vi "ToDatagram.vi"(8 "error in (no error)":errorcluster, 10 "messageID":u16, 11 "PublishReceivedMqttMsg in":refnum<class "PublishReceivedMqttMsg.lvclass">) -> (0 "error out":errorcluster, 2 "Datagram":u8[](array[numeric]), 3 "PublishReceivedMqttMsg out":refnum<class "PublishReceivedMqttMsg.lvclass">)   [LabVIEW 2020, in "PublishReceivedMqttMsg.lvclass"]
uses:
  PublishReceivedMqttMsg.lvclass
  PublishReceivedMqttMsg.lvclass/PublishReceivedMqttMsg.ctl
  mqttTypedef/MessageType.ctl
  mqttTypedef/QosLevel.ctl
  MQTT Client.lvclass
  BaseMqttMsg.lvclass
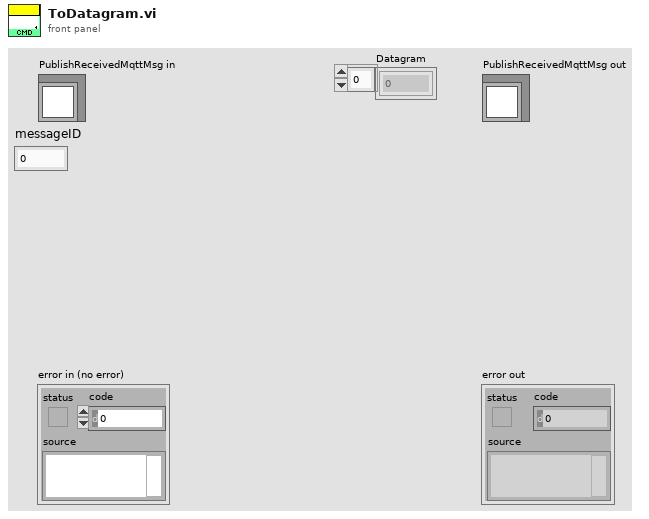
[diagram p1: front panel]
types:
  T1 = typedef "MQTT Client.lvclass/QosLevel.ctl" = enum8{"At most once", "At least once", "Exactly once", "Reserved"}
  T2 = typedef "MQTT Client.lvclass/MessageType.ctl" = enum32{"Reserved", "CONNECT", "CONNACK", "PUBLISH", "PUBACK", "PUBREC", "PUBREL", "PUBCOMP", "SUBSCRIBE", "SUBACK", "UNSUBSCRIBE", "UNSUBACK", "PINGREQ", "PINGRESP", "DISCONNECT", "Reserved2"}
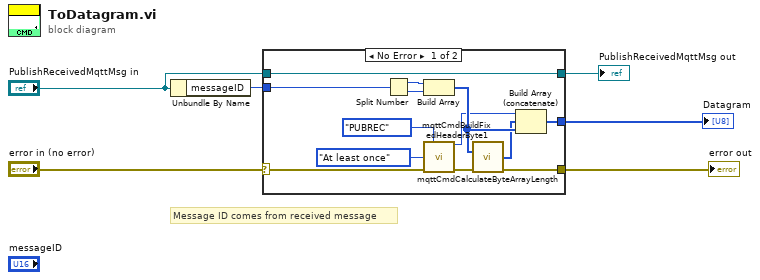
[diagram p0: block diagram]
diagram:
  # "Message ID comes from received message"
  n1 = Unbundle By Name("PublishReceivedMqttMsg in") -> ("messageID"=w6:u16)
  n2 = case shown="No Error" "error in (no error)" {
    selector: "error in (no error)" -> [w12 w21]
    tunnel: [w10 w21] -> w1
    tunnel: [w8 w20] -> w3
    tunnel: w6 -> [w9 _]
    tunnel: "PublishReceivedMqttMsg in" -> [w8 w20]
    tunnel: [w7 _] -> w4
    frame No Error {
      n3 = Split Number(x=w9) -> (hi(x)=w16:u8, lo(x)=w15:u8)
      n4 = Build Array(w16, w15) -> (w17:u8[])
      n5 = call "mqttCmdBuildFixedHeaderByte1.vi"("MessageType"=MessageType."PUBREC", "QoS (At most once)"=QosLevel."At least once", "error in (no error)"=w12) -> ("byte1"=w13:u8, "error out"=w11:errorcluster)  [unwired: 11 in]
      n6 = call "mqttCmdCalculateByteArrayLength.vi"("byteArry in"=w17, "error in (no error)"=w11) -> ("length out"=w14:u8[], "error out"=w10:errorcluster)  [unwired: 12 in]
      n7 = Build Array (concatenate)(w13, w14, w17) -> (w7:u8[])
    }
    frame Error {
    }
  }
  "error out" <- w1
  "PublishReceivedMqttMsg out" <- w3
  "Datagram" <- w4
